vi "Begin.vi"(8 "error in":errorcluster) -> (0 "error out":errorcluster)   [LabVIEW 2020]
doc: "Called before other user functions, this VI is expected to open initial I/O refnums, load in file data, and do all program initialization. Notice that the <B>error out</B> terminal is simply used for data flow. Wiring it to other structures or subVIs ensures that this VI runs first."
uses:
  <vilib>/Rock Robotics/WPI/DriverStation/WPI_DriverStationRobotMode2.ctl
  <vilib>/Rock Robotics/WPI/Joystick/WPI_JoystickDeviceEnum.ctl
  <vilib>/Rock Robotics/SystemInterfaces/i2clib/i2c_bus.ctl
  <vilib>/Rock Robotics/WPI/Solenoid/WPI_SolenoidChannel.ctl
  <vilib>/Rock Robotics/SystemInterfaces/DIO/FPGA_DIOChannel.ctl
  Robot Global Data.vi
  <vilib>/Rock Robotics/Network Tables/NT Write String Array.vi
  <vilib>/Rock Robotics/WPI/ThirdParty/Phoenix-LabVIEW/Motor Controller/Get/CTRE_Phoenix_MotorController_GetSelectedSensorData.vi
  <vilib>/Rock Robotics/WPI/Solenoid/WPI_SolenoidOpenDouble.vi
  <vilib>/Rock Robotics/WPI/Switch/WPI_SwitchOpenLimit.vi
  <vilib>/Rock Robotics/WPI/Switch/WPI_SwitchOpenCounting.vi
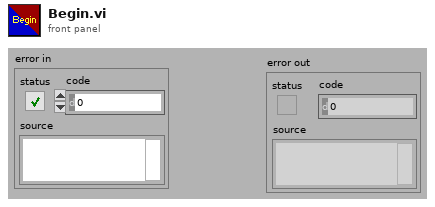
[diagram p1: front panel]
types:
  T1 = typedef "FPGA_DIOChannel.ctl" = enum8{"DIO 0", "DIO 1", "DIO 2", "DIO 3", "DIO 4", "DIO 5", "DIO 6", "DIO 7", "DIO 8", "DIO 9", "DIO MXP 0", "DIO MXP 1", "DIO MXP 2", "DIO MXP 3", "DIO MXP 4", "DIO MXP 5", "DIO MXP 6", "DIO MXP 7", "DIO MXP 8", "DIO MXP 9", "DIO MXP 10", "DIO MXP 11", "DIO MXP 12", "DIO MXP 13", "DIO MXP 14", "DIO MXP 15", "SPI Port CS1", "SPI Port CS2", "SPI Port CS3", "SPI Port MISO", "SPI Port MOSI", "Invalid"}
  T2 = typedef "WPI_SolenoidChannel.ctl" = enum8{"Solenoid 0", "Solenoid 1", "Solenoid 2", "Solenoid 3", "Solenoid 4", "Solenoid 5", "Solenoid 6", "Solenoid 7", "Solenoid 8", "Solenoid 9", "Solenoid 10", "Solenoid 11", "Solenoid 12", "Solenoid 13", "Solenoid 14", "Solenoid 15", "Invalid"}
  T3 = typedef "i2c_bus.ctl" = enum16{"I2C On-Board", "I2C MXP", "Invalid"}
  T4 = typedef "WPI_JoystickDeviceEnum.ctl" = enum16{"USB 0", "USB 1", "USB 2", "USB 3", "USB 4", "USB 5"}
  T5 = typedef "WPI_DriverStationRobotMode2.ctl" = enum16{"Autonomous Disabled", "Autonomous Enabled", "Teleop Disabled", "Teleop Enabled", "Disconnected", "Finish", "Test Disabled", "Test Enabled", "Emergency Stopped"}
  T6 = typedef "WPI_CompressorDevRef.ctl" = cluster{"DevStatus":errorcluster, "Pneumatics Control Module":u8}
  T7 = typedef "WPI_SolenoidDevRef.ctl" = cluster{"DevStatus":errorcluster, "Pneumatics Control Module":u8, "Forward Solenoid Channel":T2, "Reverse Solenoid Channel":T2}
  T8 = typedef "WPI_JoystickDevRef.ctl" = cluster{"Device":T4}
  T9 = typedef "WPI_MotorControlDeviceRef.ctl" = cluster{"DeviceStatus":errorcluster, "Type":T10, "PWM":cluster{"PWM Channel":T11, "DeadBand":T12}, "CAN":cluster{"Device Number":u8, "SetOutput VI Ref":variant, "GetOutput VI Ref":variant, "Enable VI Ref":variant, "Disable VI Ref":variant, "Data":variant}, "Invert":bool, "DIO PWM":cluster{"PWM \"Enable\" Channel":T11, "DIOChannel":T1, "PWM Rate":dbl}}
  T10 = typedef "WPI_MotorControlType.ctl" = enum16{"PWM", "CAN", "DIO PWM"}
  T11 = typedef "FPGA_DIOPWMChannel.ctl" = enum8{"PWM 0", "PWM 1", "PWM 2", "PWM 3", "PWM 4", "PWM 5", "PWM 6", "PWM 7", "PWM 8", "PWM 9", "PWM MXP 0", "PWM MXP 1", "PWM MXP 2", "PWM MXP 3", "PWM MXP 4", "PWM MXP 5", "PWM MXP 6", "PWM MXP 7", "PWM MXP 8", "PWM MXP 9", "Invalid"}
  T12 = typedef "WPI_PWMDeadband.ctl" = cluster{"Name":string, "maxPositivePwm":i32, "minPositivePwm":i32, "centerPwm":i32, "maxNegativePwm":i32, "minNegativePwm":i32, "angularRange":u16}
  T13 = typedef "Color Sensor V3 DevRef.ctl" = cluster{"I2CDevRef":T14}
  T14 = typedef "WPI_I2CDevRef.ctl" = cluster{"DevStatus":errorcluster, "Device Address":u8, "Handle":i32, "I2C Bus":T3}
  T15 = typedef "CTRE_PigeonIMU_DeviceRef.ctl" = cluster{"DeviceStatus":errorcluster, "Device Number":u8, "Type":T16, "Device ID":u32, "Handle":u64, "UsageFrame":u32, "Library Path":path}
  T16 = typedef "CTRE_PigeonIMU_ConnectionType.ctl" = u32
  T17 = typedef "CTRE_Phoenix_CANcoder_DeviceRef.ctl" = cluster{"DeviceStatus":errorcluster, "Device Number":u8, "Handle":u64, "UsageFrame":u32, "Library Path":path}
  T18 = typedef "WPI_SwitchDevRef.ctl" = cluster{"DevStatus":errorcluster, "DIO Channel":T1, "CntIndex":T19, "Normally Closed":bool}
  T19 = typedef "FPGA_CounterCtrSystemIndex.ctl" = enum8{"Ctr 0", "Ctr 1", "Ctr 2", "Ctr 3", "Ctr 4", "Ctr 5", "Ctr 6", "Ctr 7", "Invalid"}
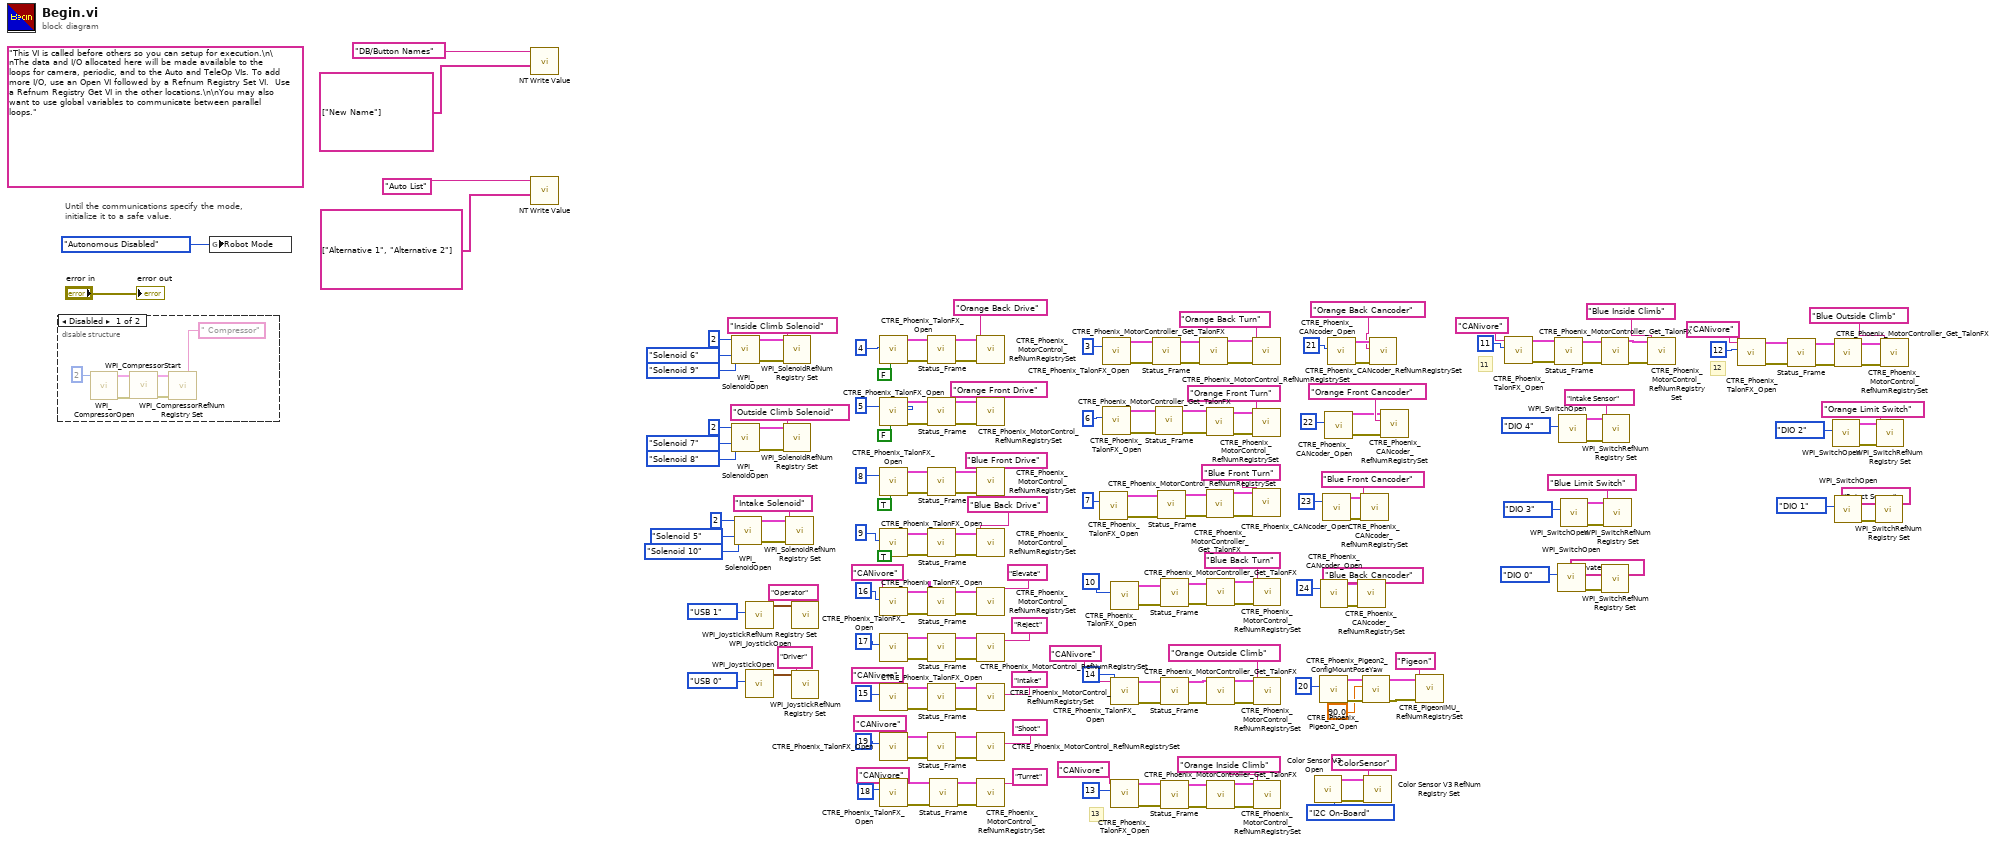
[diagram p0: block diagram]
diagram:
  (unwired) "This VI is called before others so you can setup for execution.\n\nThe data and I/O allocated here will be made available to the loops for camera, periodic, and to the Auto and TeleOp VIs. To add more I/O, use an Open VI followed by a Refnum Registry Set VI.  Use a Refnum Registry Get VI in the other locations.\n\nYou may also want to use global variables to communicate between parallel loops."
  # "13"
  # "12"
  # "11"
  # "Until the communications specify the mode,\ninitialize it to a safe value."
  n1 = disable-structure shown="Disabled" {
    frame Disabled {
      n2 = call <vilib>:"WPI_CompressorOpen.vi"("Pneumatics device (def)"=u8 2) -> ("CompressorDevRef"=w212:T6, "error out"=w213:errorcluster)  [unwired: 13 in]
      n3 = call <vilib>:"WPI_CompressorStart.vi"("error in (no error)"=w213, "CompressorDevRef"=w212) -> ("error out"=w211:errorcluster, "CompressorDevRef"=w210:T6)  [unwired: 8 in]
      n4 = call <vilib>:"WPI_CompressorRefNum Registry Set.vi"("error in (no error)"=w211, "refnum name"=" Compressor", "CompressorDevRef"=w210) -> ()  [unwired: 7 in, 2 out]
    }
    frame Enabled {
    }
  }
  n5 = global write "Robot Global Data.vi" "Robot Mode"(WPI_DriverStationRobotMode2."Autonomous Disabled" ("Robot Mode")) -> ()
  n6 = call-poly <vilib>:"NT Write Value.vi"("String Array"=string[] ["New Name"], "Name"="DB/Button Names") -> ()  [unwired: 9 in, 1 out]
  n7 = call-poly <vilib>:"NT Write Value.vi"("String Array"=string[] ["Alternative 1", "Alternative 2"], "Name"="Auto List") -> ()  [unwired: 9 in, 1 out]
  n8 = call-poly <vilib>:"WPI_SolenoidOpen.vi"("Reverse Solenoid Channel"=WPI_SolenoidChannel."Solenoid 9", "Forward Solenoid Channel"=WPI_SolenoidChannel."Solenoid 6", "Pneumatics Device (def)"=u8 2) -> ("error out"=w156:errorcluster, "SolenoidDevRef"=w155:T7)  [unwired: 7 in]
  n9 = call-poly <vilib>:"WPI_SolenoidOpen.vi"("Reverse Solenoid Channel"=WPI_SolenoidChannel."Solenoid 8", "Forward Solenoid Channel"=WPI_SolenoidChannel."Solenoid 7", "Pneumatics Device (def)"=u8 2) -> ("error out"=w153:errorcluster, "SolenoidDevRef"=w152:T7)  [unwired: 7 in]
  n10 = call-poly <vilib>:"WPI_SolenoidOpen.vi"("Reverse Solenoid Channel"=WPI_SolenoidChannel."Solenoid 10", "Forward Solenoid Channel"=WPI_SolenoidChannel."Solenoid 5", "Pneumatics Device (def)"=u8 2) -> ("error out"=w150:errorcluster, "SolenoidDevRef"=w149:T7)  [unwired: 7 in]
  n11 = call <vilib>:"WPI_JoystickOpen.vi"("JoystickDevice"=WPI_JoystickDeviceEnum."USB 1") -> ("JoystickDevRef"=w197:T8)  [unwired: 10 in]
  n12 = call <vilib>:"WPI_JoystickOpen.vi"("JoystickDevice"=WPI_JoystickDeviceEnum."USB 0") -> ("JoystickDevRef"=w205:T8)  [unwired: 10 in]
  n13 = call <vilib>:"WPI_SolenoidRefNum Registry Set.vi"("error in (no error)"=w156, "refnum name"="Inside Climb Solenoid", "SolenoidDevRef"=w155) -> ()  [unwired: 7 in, 2 out]
  n14 = call <vilib>:"WPI_SolenoidRefNum Registry Set.vi"("error in (no error)"=w153, "refnum name"="Outside Climb Solenoid", "SolenoidDevRef"=w152) -> ()  [unwired: 7 in, 2 out]
  n15 = call <vilib>:"WPI_SolenoidRefNum Registry Set.vi"("error in (no error)"=w150, "refnum name"="Intake Solenoid", "SolenoidDevRef"=w149) -> ()  [unwired: 7 in, 2 out]
  n16 = call <vilib>:"WPI_JoystickRefNum Registry Set.vi"("refnum name"="Operator", "JoystickDevRef"=w197) -> ()  [unwired: 8 in, 2 out]
  n17 = call <vilib>:"WPI_JoystickRefNum Registry Set.vi"("refnum name"="Driver", "JoystickDevRef"=w205) -> ()  [unwired: 8 in, 2 out]
  n18 = call <vilib>:"CTRE_Phoenix_TalonFX_Open.vi"("Invert"=FALSE, "Device Number"=u8 4) -> ("error out"=w71:errorcluster, "PhoenixMotorControlDevRef"=w72:T9)  [unwired: 8 in]
  n19 = call <vilib>:"CTRE_Phoenix_TalonFX_Open.vi"("Invert"=FALSE, "Device Number"=u8 5) -> ("error out"=w64:errorcluster, "PhoenixMotorControlDevRef"=w63:T9)  [unwired: 8 in]
  n20 = call <vilib>:"CTRE_Phoenix_TalonFX_Open.vi"("Invert"=TRUE, "Device Number"=u8 8) -> ("error out"=w68:errorcluster, "PhoenixMotorControlDevRef"=w65:T9)  [unwired: 8 in]
  n21 = call <vilib>:"CTRE_Phoenix_TalonFX_Open.vi"("Invert"=TRUE, "Device Number"=u8 9) -> ("error out"=w57:errorcluster, "PhoenixMotorControlDevRef"=w60:T9)  [unwired: 8 in]
  n22 = call <vilib>:"CTRE_Phoenix_TalonFX_Open.vi"("Device Number"=u8 16, "CAN Bus"="CANivore") -> ("error out"=w53:errorcluster, "PhoenixMotorControlDevRef"=w56:T9)  [unwired: 8 in]
  n23 = call <vilib>:"CTRE_Phoenix_TalonFX_Open.vi"("Device Number"=u8 17) -> ("error out"=w49:errorcluster, "PhoenixMotorControlDevRef"=w52:T9)  [unwired: 9 in]
  n24 = call <vilib>:"CTRE_Phoenix_TalonFX_Open.vi"("Device Number"=u8 15, "CAN Bus"="CANivore") -> ("error out"=w45:errorcluster, "PhoenixMotorControlDevRef"=w48:T9)  [unwired: 8 in]
  n25 = call <vilib>:"CTRE_Phoenix_TalonFX_Open.vi"("Device Number"=u8 19, "CAN Bus"="CANivore") -> ("error out"=w41:errorcluster, "PhoenixMotorControlDevRef"=w44:T9)  [unwired: 8 in]
  n26 = call <vilib>:"CTRE_Phoenix_TalonFX_Open.vi"("Device Number"=u8 18, "CAN Bus"="CANivore") -> ("error out"=w36:errorcluster, "PhoenixMotorControlDevRef"=w39:T9)  [unwired: 8 in]
  n27 = call "Status_Frame.vi"("error in (no error)"=w71, "Motor Control DevRef"=w72) -> ("error out"=w70:errorcluster, "PhoenixMotorControlDevRef"=w69:T9)  [unwired: 8 in]
  n28 = call "Status_Frame.vi"("error in (no error)"=w64, "Motor Control DevRef"=w63) -> ("error out"=w61:errorcluster, "PhoenixMotorControlDevRef"=w62:T9)  [unwired: 8 in]
  n29 = call "Status_Frame.vi"("error in (no error)"=w68, "Motor Control DevRef"=w65) -> ("error out"=w67:errorcluster, "PhoenixMotorControlDevRef"=w66:T9)  [unwired: 8 in]
  n30 = call "Status_Frame.vi"("error in (no error)"=w57, "Motor Control DevRef"=w60) -> ("error out"=w58:errorcluster, "PhoenixMotorControlDevRef"=w59:T9)  [unwired: 8 in]
  n31 = call "Status_Frame.vi"("error in (no error)"=w53, "Motor Control DevRef"=w56) -> ("error out"=w54:errorcluster, "PhoenixMotorControlDevRef"=w55:T9)  [unwired: 8 in]
  n32 = call "Status_Frame.vi"("error in (no error)"=w49, "Motor Control DevRef"=w52) -> ("error out"=w50:errorcluster, "PhoenixMotorControlDevRef"=w51:T9)  [unwired: 8 in]
  n33 = call "Status_Frame.vi"("error in (no error)"=w45, "Motor Control DevRef"=w48) -> ("error out"=w46:errorcluster, "PhoenixMotorControlDevRef"=w47:T9)  [unwired: 8 in]
  n34 = call "Status_Frame.vi"("error in (no error)"=w41, "Motor Control DevRef"=w44) -> ("error out"=w42:errorcluster, "PhoenixMotorControlDevRef"=w43:T9)  [unwired: 8 in]
  n35 = call "Status_Frame.vi"("error in (no error)"=w36, "Motor Control DevRef"=w39) -> ("error out"=w37:errorcluster, "PhoenixMotorControlDevRef"=w38:T9)  [unwired: 8 in]
  n36 = call <vilib>:"CTRE_Phoenix_MotorControl_RefNumRegistrySet.vi"("error in (no error)"=w70, "refnum name"="Orange Back Drive", "PhoenixMotorControlDevRef"=w69) -> ()  [unwired: 7 in, 2 out]
  n37 = call <vilib>:"CTRE_Phoenix_MotorControl_RefNumRegistrySet.vi"("error in (no error)"=w61, "refnum name"="Orange Front Drive", "PhoenixMotorControlDevRef"=w62) -> ()  [unwired: 7 in, 2 out]
  n38 = call <vilib>:"CTRE_Phoenix_MotorControl_RefNumRegistrySet.vi"("error in (no error)"=w67, "refnum name"="Blue Front Drive", "PhoenixMotorControlDevRef"=w66) -> ()  [unwired: 7 in, 2 out]
  n39 = call <vilib>:"CTRE_Phoenix_MotorControl_RefNumRegistrySet.vi"("error in (no error)"=w58, "refnum name"="Blue Back Drive", "PhoenixMotorControlDevRef"=w59) -> ()  [unwired: 7 in, 2 out]
  n40 = call <vilib>:"CTRE_Phoenix_MotorControl_RefNumRegistrySet.vi"("error in (no error)"=w54, "refnum name"="Elevate", "PhoenixMotorControlDevRef"=w55) -> ()  [unwired: 7 in, 2 out]
  n41 = call <vilib>:"CTRE_Phoenix_MotorControl_RefNumRegistrySet.vi"("error in (no error)"=w50, "refnum name"="Reject", "PhoenixMotorControlDevRef"=w51) -> ()  [unwired: 7 in, 2 out]
  n42 = call <vilib>:"CTRE_Phoenix_MotorControl_RefNumRegistrySet.vi"("error in (no error)"=w46, "refnum name"="Intake", "PhoenixMotorControlDevRef"=w47) -> ()  [unwired: 7 in, 2 out]
  n43 = call <vilib>:"CTRE_Phoenix_MotorControl_RefNumRegistrySet.vi"("error in (no error)"=w42, "refnum name"="Shoot", "PhoenixMotorControlDevRef"=w43) -> ()  [unwired: 7 in, 2 out]
  n44 = call <vilib>:"CTRE_Phoenix_MotorControl_RefNumRegistrySet.vi"("error in (no error)"=w37, "refnum name"="Turret", "PhoenixMotorControlDevRef"=w38) -> ()  [unwired: 7 in, 2 out]
  n45 = call <vilib>:"CTRE_Phoenix_TalonFX_Open.vi"("Device Number"=u8 7) -> ("error out"=w24:errorcluster, "PhoenixMotorControlDevRef"=w27:T9)  [unwired: 9 in]
  n46 = call <vilib>:"CTRE_Phoenix_TalonFX_Open.vi"("Device Number"=u8 3) -> ("error out"=w32:errorcluster, "PhoenixMotorControlDevRef"=w35:T9)  [unwired: 9 in]
  n47 = call <vilib>:"CTRE_Phoenix_TalonFX_Open.vi"("Device Number"=u8 6) -> ("error out"=w28:errorcluster, "PhoenixMotorControlDevRef"=w31:T9)  [unwired: 9 in]
  n48 = call <vilib>:"CTRE_Phoenix_TalonFX_Open.vi"("Device Number"=u8 10) -> ("error out"=w20:errorcluster, "PhoenixMotorControlDevRef"=w21:T9)  [unwired: 9 in]
  n49 = call <vilib>:"CTRE_Phoenix_TalonFX_Open.vi"("Device Number"=u8 14, "CAN Bus"="CANivore") -> ("error out"=w10:errorcluster, "PhoenixMotorControlDevRef"=w11:T9)  [unwired: 8 in]
  n50 = call <vilib>:"CTRE_Phoenix_TalonFX_Open.vi"("Device Number"=u8 13, "CAN Bus"="CANivore") -> ("error out"=w8:errorcluster, "PhoenixMotorControlDevRef"=w9:T9)  [unwired: 8 in]
  n51 = call "Status_Frame.vi"("error in (no error)"=w32, "Motor Control DevRef"=w35) -> ("error out"=w33:errorcluster, "PhoenixMotorControlDevRef"=w34:T9)  [unwired: 8 in]
  n52 = call "Status_Frame.vi"("error in (no error)"=w28, "Motor Control DevRef"=w31) -> ("error out"=w29:errorcluster, "PhoenixMotorControlDevRef"=w30:T9)  [unwired: 8 in]
  n53 = call "Status_Frame.vi"("error in (no error)"=w24, "Motor Control DevRef"=w27) -> ("error out"=w25:errorcluster, "PhoenixMotorControlDevRef"=w26:T9)  [unwired: 8 in]
  n54 = call "Status_Frame.vi"("error in (no error)"=w20, "Motor Control DevRef"=w21) -> ("error out"=w22:errorcluster, "PhoenixMotorControlDevRef"=w23:T9)  [unwired: 8 in]
  n55 = call "Status_Frame.vi"("error in (no error)"=w10, "Motor Control DevRef"=w11) -> ("error out"=w18:errorcluster, "PhoenixMotorControlDevRef"=w19:T9)  [unwired: 8 in]
  n56 = call "Status_Frame.vi"("error in (no error)"=w8, "Motor Control DevRef"=w9) -> ("error out"=w16:errorcluster, "PhoenixMotorControlDevRef"=w17:T9)  [unwired: 8 in]
  n57 = call-poly <vilib>:"CTRE_Phoenix_MotorController_Get_TalonFX.vi"("PhoenixMotorControlDevRef"=w34, "error in"=w33) -> ("PhoenixMotorControlDevRef"=w93:T9, "error out"=w195:errorcluster)  [unwired: 10 in, 2 out]
  n58 = call-poly <vilib>:"CTRE_Phoenix_MotorController_Get_TalonFX.vi"("PhoenixMotorControlDevRef"=w30, "error in"=w29) -> ("PhoenixMotorControlDevRef"=w188:T9, "error out"=w189:errorcluster)  [unwired: 10 in, 2 out]
  n59 = call-poly <vilib>:"CTRE_Phoenix_MotorController_Get_TalonFX.vi"("PhoenixMotorControlDevRef"=w26, "error in"=w25) -> ("PhoenixMotorControlDevRef"=w99:T9, "error out"=w94:errorcluster)  [unwired: 10 in, 2 out]
  n60 = call-poly <vilib>:"CTRE_Phoenix_MotorController_Get_TalonFX.vi"("PhoenixMotorControlDevRef"=w23, "error in"=w22) -> ("PhoenixMotorControlDevRef"=w95:T9, "error out"=w176:errorcluster)  [unwired: 10 in, 2 out]
  n61 = call-poly <vilib>:"CTRE_Phoenix_MotorController_Get_TalonFX.vi"("PhoenixMotorControlDevRef"=w19, "error in"=w18) -> ("PhoenixMotorControlDevRef"=w96:T9, "error out"=w113:errorcluster)  [unwired: 10 in, 2 out]
  n62 = call-poly <vilib>:"CTRE_Phoenix_MotorController_Get_TalonFX.vi"("PhoenixMotorControlDevRef"=w17, "error in"=w16) -> ("PhoenixMotorControlDevRef"=w98:T9, "error out"=w110:errorcluster)  [unwired: 10 in, 2 out]
  n63 = call <vilib>:"CTRE_Phoenix_MotorControl_RefNumRegistrySet.vi"("error in (no error)"=w195, "refnum name"="Orange Back Turn", "PhoenixMotorControlDevRef"=w93) -> ()  [unwired: 7 in, 2 out]
  n64 = call <vilib>:"CTRE_Phoenix_MotorControl_RefNumRegistrySet.vi"("error in (no error)"=w189, "refnum name"="Orange Front Turn", "PhoenixMotorControlDevRef"=w188) -> ()  [unwired: 7 in, 2 out]
  n65 = call <vilib>:"CTRE_Phoenix_MotorControl_RefNumRegistrySet.vi"("error in (no error)"=w94, "refnum name"="Blue Front Turn", "PhoenixMotorControlDevRef"=w99) -> ()  [unwired: 7 in, 2 out]
  n66 = call <vilib>:"CTRE_Phoenix_MotorControl_RefNumRegistrySet.vi"("error in (no error)"=w176, "refnum name"="Blue Back Turn", "PhoenixMotorControlDevRef"=w95) -> ()  [unwired: 7 in, 2 out]
  n67 = call <vilib>:"CTRE_Phoenix_MotorControl_RefNumRegistrySet.vi"("error in (no error)"=w113, "refnum name"="Orange Outside Climb", "PhoenixMotorControlDevRef"=w96) -> ()  [unwired: 7 in, 2 out]
  n68 = call <vilib>:"CTRE_Phoenix_MotorControl_RefNumRegistrySet.vi"("error in (no error)"=w110, "refnum name"="Orange Inside Climb", "PhoenixMotorControlDevRef"=w98) -> ()  [unwired: 7 in, 2 out]
  n69 = call <vilib>:"Color Sensor V3 Open.vi"("I2C Bus"=i2c_bus."I2C On-Board") -> ("error out"=w160:errorcluster, "ColorSensorDevRef"=w159:T13)  [unwired: 9 in]
  n70 = call <vilib>:"CTRE_Phoenix_Pigeon2_Open.vi"("Device Number"=u8 20) -> ("error out"=w86:errorcluster, "PigeonIMUDevRef"=w87:T15)  [unwired: 9 in]
  n71 = call <vilib>:"CTRE_Phoenix_CANcoder_Open.vi"("Device Number"=u8 24) -> ("error out"=w88:errorcluster, "CTRE_CANcoder_DeviceRef"=w89:T17)  [unwired: 9 in]
  n72 = call <vilib>:"CTRE_Phoenix_CANcoder_Open.vi"("Device Number"=u8 23) -> ("error out"=w90:errorcluster, "CTRE_CANcoder_DeviceRef"=w91:T17)  [unwired: 9 in]
  n73 = call <vilib>:"CTRE_Phoenix_CANcoder_Open.vi"("Device Number"=u8 22) -> ("error out"=w82:errorcluster, "CTRE_CANcoder_DeviceRef"=w81:T17)  [unwired: 9 in]
  n74 = call <vilib>:"CTRE_Phoenix_CANcoder_Open.vi"("Device Number"=u8 21) -> ("error out"=w2:errorcluster, "CTRE_CANcoder_DeviceRef"=w3:T17)  [unwired: 9 in]
  n75 = call <vilib>:"CTRE_Phoenix_CANcoder_RefNumRegistrySet.vi"("error in (no error)"=w88, "refnum name"="Blue Back Cancoder", "CTRE_CANcoder_DeviceRef"=w89) -> ()  [unwired: 7 in, 2 out]
  n76 = call <vilib>:"CTRE_Phoenix_CANcoder_RefNumRegistrySet.vi"("error in (no error)"=w90, "refnum name"="Blue Front Cancoder", "CTRE_CANcoder_DeviceRef"=w91) -> ()  [unwired: 7 in, 2 out]
  n77 = call <vilib>:"CTRE_Phoenix_Pigeon2_ConfigMountPoseYaw.vi"("error in"=w86, "Yaw"=90.0, "PigeonIMUDevRef"=w87) -> ("error out"=w84:errorcluster, "PigeonIMUDevRef 2"=w85:T15)  [unwired: 7 in]
  n78 = call <vilib>:"Color Sensor V3 RefNum Registry Set.vi"("error in (no error)"=w160, "refnum name"="ColorSensor", "ColorSensorDevRef"=w159) -> ()  [unwired: 7 in, 2 out]
  n79 = call <vilib>:"CTRE_Phoenix_CANcoder_RefNumRegistrySet.vi"("error in (no error)"=w2, "refnum name"="Orange Back Cancoder", "CTRE_CANcoder_DeviceRef"=w3) -> ()  [unwired: 7 in, 2 out]
  n80 = call <vilib>:"CTRE_Phoenix_CANcoder_RefNumRegistrySet.vi"("error in (no error)"=w82, "refnum name"="Orange Front Cancoder", "CTRE_CANcoder_DeviceRef"=w81) -> ()  [unwired: 7 in, 2 out]
  n81 = call <vilib>:"CTRE_PigeonIMU_RefNumRegistrySet.vi"("error in (no error)"=w84, "refnum name"="Pigeon", "PigeonIMUDevRef"=w85) -> ()  [unwired: 7 in, 2 out]
  n82 = call <vilib>:"CTRE_Phoenix_TalonFX_Open.vi"("Device Number"=u8 11, "CAN Bus"="CANivore") -> ("error out"=w4:errorcluster, "PhoenixMotorControlDevRef"=w5:T9)  [unwired: 8 in]
  n83 = call "Status_Frame.vi"("error in (no error)"=w4, "Motor Control DevRef"=w5) -> ("error out"=w12:errorcluster, "PhoenixMotorControlDevRef"=w13:T9)  [unwired: 8 in]
  n84 = call-poly <vilib>:"WPI_SwitchOpen.vi"("DIO Channel"=FPGA_DIOChannel."DIO 0") -> ("error out"=w138:errorcluster, "SwitchDevRef"=w137:T18)  [unwired: 9 in]
  n85 = call-poly <vilib>:"WPI_SwitchOpen.vi"("DIO Channel"=FPGA_DIOChannel."DIO 4") -> ("error out"=w117:errorcluster, "SwitchDevRef"=w116:T18)  [unwired: 9 in]
  n86 = call-poly <vilib>:"WPI_SwitchOpen.vi"("DIO Channel"=FPGA_DIOChannel."DIO 3") -> ("error out"=w121:errorcluster, "SwitchDevRef"=w120:T18)  [unwired: 9 in]
  n87 = call-poly <vilib>:"CTRE_Phoenix_MotorController_Get_TalonFX.vi"("PhoenixMotorControlDevRef"=w13, "error in"=w12) -> ("PhoenixMotorControlDevRef"=w102:T9, "error out"=w103:errorcluster)  [unwired: 10 in, 2 out]
  n88 = call <vilib>:"WPI_SwitchRefNum Registry Set.vi"("error in (no error)"=w138, "refnum name"="Elevate Sensor", "SwitchDevRef"=w137) -> ()  [unwired: 7 in, 2 out]
  n89 = call <vilib>:"WPI_SwitchRefNum Registry Set.vi"("error in (no error)"=w117, "refnum name"="Intake Sensor", "SwitchDevRef"=w116) -> ()  [unwired: 7 in, 2 out]
  n90 = call <vilib>:"WPI_SwitchRefNum Registry Set.vi"("error in (no error)"=w121, "refnum name"="Blue Limit Switch", "SwitchDevRef"=w120) -> ()  [unwired: 7 in, 2 out]
  n91 = call <vilib>:"CTRE_Phoenix_MotorControl_RefNumRegistrySet.vi"("error in (no error)"=w103, "refnum name"="Blue Inside Climb", "PhoenixMotorControlDevRef"=w102) -> ()  [unwired: 7 in, 2 out]
  n92 = call <vilib>:"CTRE_Phoenix_TalonFX_Open.vi"("Device Number"=u8 12, "CAN Bus"="CANivore") -> ("error out"=w6:errorcluster, "PhoenixMotorControlDevRef"=w7:T9)  [unwired: 8 in]
  n93 = call "Status_Frame.vi"("error in (no error)"=w6, "Motor Control DevRef"=w7) -> ("error out"=w14:errorcluster, "PhoenixMotorControlDevRef"=w15:T9)  [unwired: 8 in]
  n94 = call-poly <vilib>:"WPI_SwitchOpen.vi"("DIO Channel"=FPGA_DIOChannel."DIO 2") -> ("error out"=w125:errorcluster, "SwitchDevRef"=w124:T18)  [unwired: 9 in]
  n95 = call-poly <vilib>:"CTRE_Phoenix_MotorController_Get_TalonFX.vi"("PhoenixMotorControlDevRef"=w15, "error in"=w14) -> ("PhoenixMotorControlDevRef"=w106:T9, "error out"=w107:errorcluster)  [unwired: 10 in, 2 out]
  n96 = call-poly <vilib>:"WPI_SwitchOpen.vi"("DIO Channel"=FPGA_DIOChannel."DIO 1") -> ("error out"=w134:errorcluster, "SwitchDevRef"=w133:T18)  [unwired: 9 in]
  n97 = call <vilib>:"WPI_SwitchRefNum Registry Set.vi"("error in (no error)"=w134, "refnum name"="Reject Sensor", "SwitchDevRef"=w133) -> ()  [unwired: 7 in, 2 out]
  n98 = call <vilib>:"WPI_SwitchRefNum Registry Set.vi"("error in (no error)"=w125, "refnum name"="Orange Limit Switch", "SwitchDevRef"=w124) -> ()  [unwired: 7 in, 2 out]
  n99 = call <vilib>:"CTRE_Phoenix_MotorControl_RefNumRegistrySet.vi"("error in (no error)"=w107, "refnum name"="Blue Outside Climb", "PhoenixMotorControlDevRef"=w106) -> ()  [unwired: 7 in, 2 out]
  "error out" <- "error in"
